vi "OtmMain.vi"() -> ()   [LabVIEW 2017]
doc: "This Continuous Measurement sample project is based on the Queued Message Handler template.\n\nThe Event Handling Loop generates messages based on user interface actions.\n\nThe Message Handling Loop processes messages generated by the Event Handling Loop, or by other messages. There are also Acquisition and Logging message handling loop subVIs, and a chart updating loop."
uses:
  Settings/Settings.ctl
  Acquisition/Hardware Configuration.ctl
  Acquisition/Signal Type.ctl
  Logging/Logging Configuration.ctl
  controls/UI Data.ctl
  controls/UI State.ctl
  support/Message Queue/Enqueue Message (Single).vi
  support/Message Queue/Enqueue Message (Array).vi
  <vilib>/Utility/error.llb/Error Cluster From Error Code.vi
  <vilib>/ErrorRing/Error Ring.xnode
  Logging/Logging.lvlib
  Settings/Settings.lvlib
  Acquisition/Acquisition.lvlib
  support/User Event - Stop/User Event - Stop.lvlib
  support/Message Queue/Message Queue.lvlib
  Settings/Settings Dialog.vi
panel:
  out "Data":waveform(dbl)[](graph)
  in  "Settings":bool
  in  "Start":bool
  in  "Stop":bool
  out "Status":string
  in  "Exit":bool
  # "Continuous Measurement Data Logger"
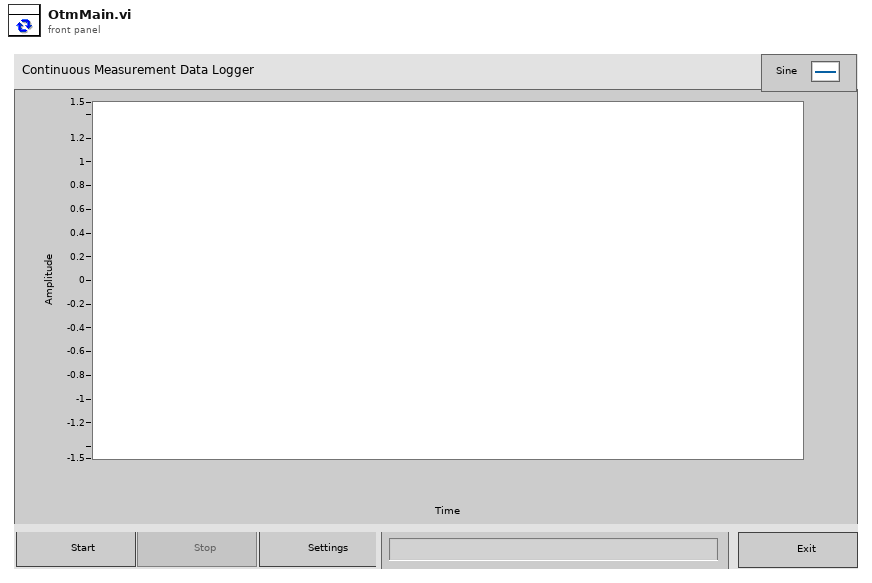
[diagram p1: front panel]
types:
  T1 = typedef "UI State.ctl" = enum16{"Idle", "Acquiring and Logging", "Waiting for Exit", "Waiting for Exit (Acq Stopped)", "Waiting for Exit (Log Stopped)", "Waiting for Stop", "Waiting for Stop (Acq Stopped)", "Waiting for Stop (Log Stopped)"}
  T2 = typedef "UI Data.ctl" = cluster{"Start Ref":refnum<vi>, "Stop Ref":refnum<vi>, "Settings Ref":refnum<vi>, "Exit Ref":refnum<vi>, "Status Ref":refnum<vi>, "Data Ref":refnum<vi>}
  T3 = typedef "Settings.lvlib/Settings.ctl" = cluster{"Hardware Configuration":T4, "Logging Configuration":T6}
  T4 = typedef "Acquisition.lvlib/Hardware Configuration.ctl" = cluster{"HW Refnum <Replace Me>":string, "Signal Type <Replace Me>":T5}
  T5 = typedef "Acquisition.lvlib/Signal Type.ctl" = enum16{"Sine Wave", "Square with Noise"}
  T6 = typedef "Logging.lvlib/Logging Configuration.ctl" = cluster{"Log File Base Path":path, "TDMS File Reference":refnum<k34>}
  T7 = typedef "Message Queue.lvlib/All Message Queues.ctl" = cluster{"UI":refnum<queue>, "Acquisition":refnum<queue>, "Logging":refnum<queue>}
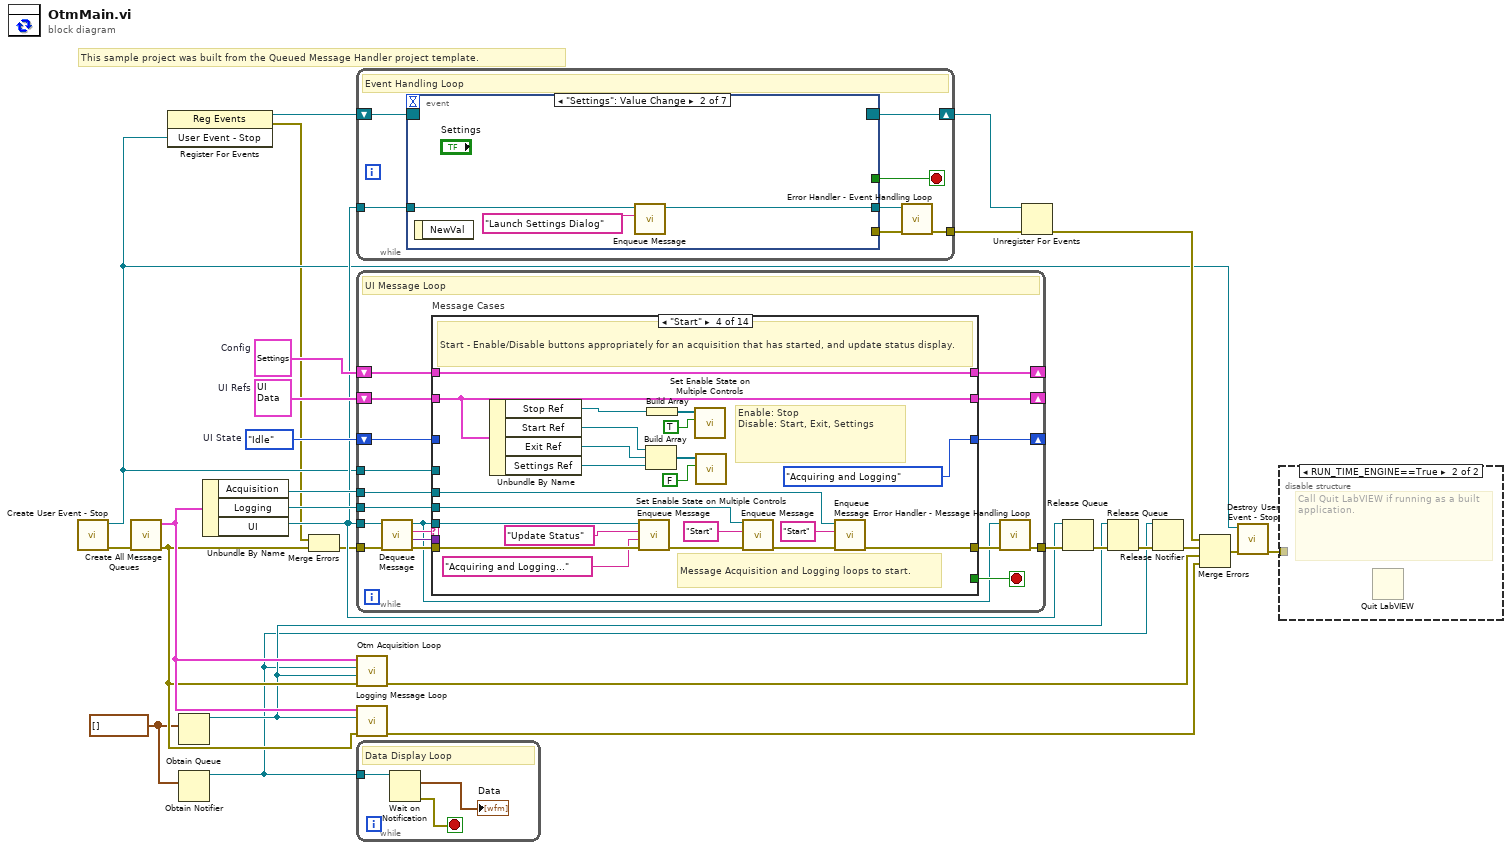
[diagram p0: block diagram]
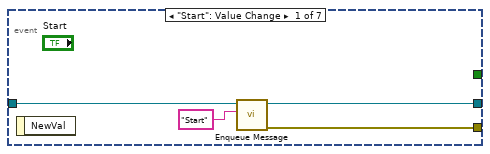
[diagram p3: hidden frame]
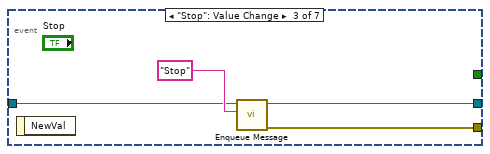
[diagram p4: hidden frame]
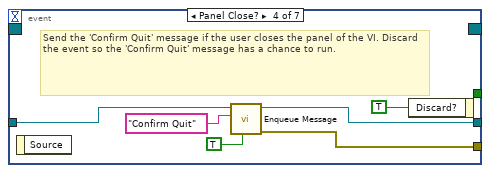
[diagram p5: hidden frame]
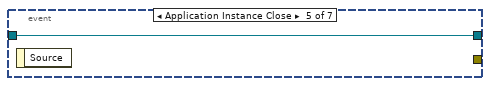
[diagram p6: hidden frame]
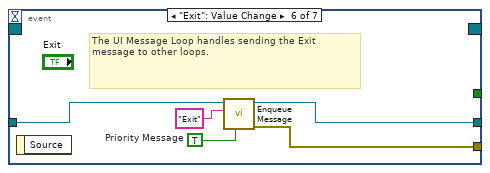
[diagram p7: hidden frame]
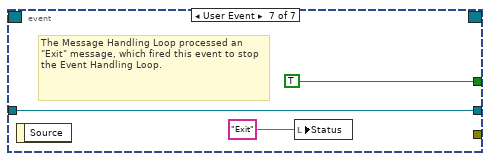
[diagram p8: hidden frame]
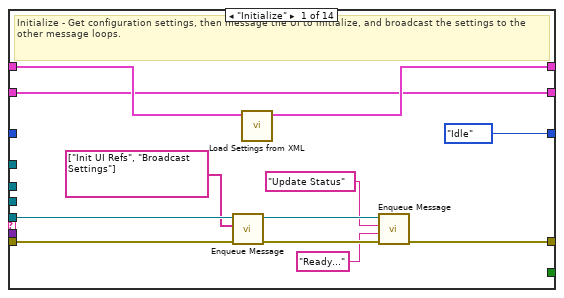
[diagram p9: hidden frame]
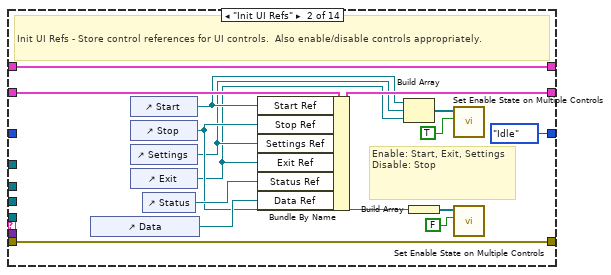
[diagram p10: hidden frame]
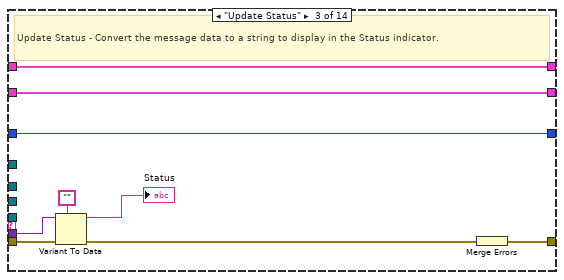
[diagram p11: hidden frame]
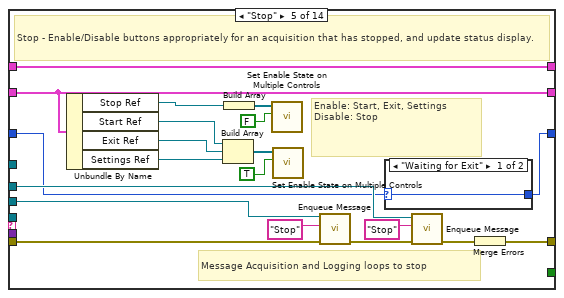
[diagram p12: hidden frame]
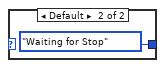
[diagram p13: hidden frame]
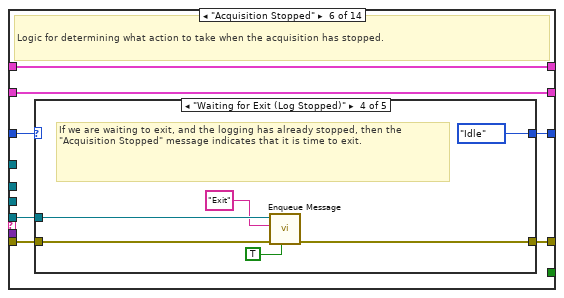
[diagram p14: hidden frame]
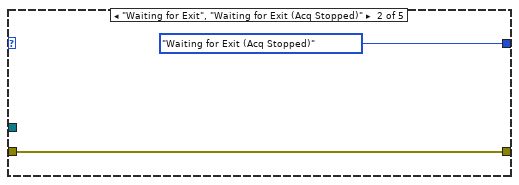
[diagram p16: hidden frame]
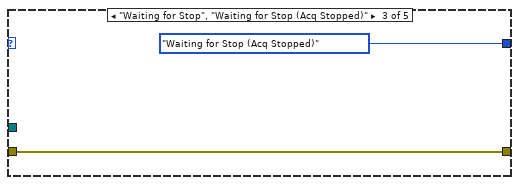
[diagram p17: hidden frame]
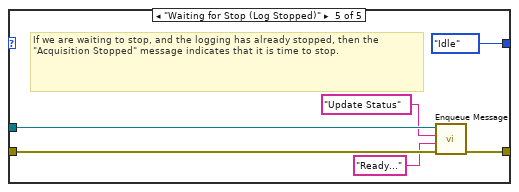
[diagram p18: hidden frame]
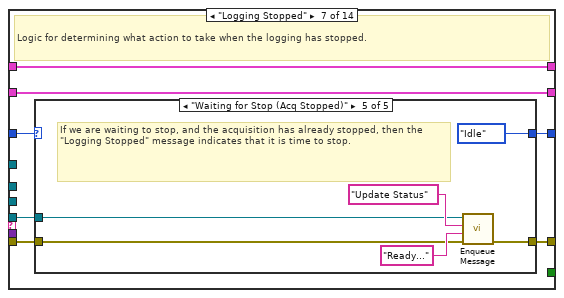
[diagram p19: hidden frame]
diagram:
  w14 = UI_State."Idle"  # UI State
  w5 = waveform(dbl)[] []
  w17 = T2 {"Start Ref"=refnum, "Stop Ref"=refnum, "Settings Ref"=refnum, "Exit Ref"=refnum, "Status Ref"=refnum, "Data Ref"=refnum}  # UI Refs
  w20 = T3 {"Hardware Configuration"={"HW Refnum <Replace Me>"="", "Signal Type <Replace Me>"=enum."Sine Wave"}, "Logging Configuration"={"Log File Base Path"=path "", "TDMS File Reference"=refnum}}  # Config
  # "This sample project was built from the Queued Message Handler project template."
  n1 = call "Create User Event - Stop.vi"() -> ("error out"=w24:errorcluster, "User Event - Stop"=w3:refnum<user-event>)  [unwired: 10 in]
  n2 = call "Create All Message Queues.vi"("error in (no error)"=w24) -> ("error out"=w21:errorcluster, "Message Queues out"=w23:T7)  [unwired: 9 in]
  n3 = register-events(w3) -> (reference out=w4:refnum<event-registration>, error out=w1:errorcluster)  [unwired: 2 in]
  n4 = Obtain Queue(element data type=w5) -> (queue out=w7:refnum<queue>)  [unwired: 4 in, 2 out]
  n5 = Obtain Notifier(notification data type=w5) -> (notifier out=w6:refnum<notifier>)  [unwired: 3 in, 2 out]
  n6 = Unbundle By Name(w23) -> ("Acquisition"=w16:refnum<queue>, "Logging"=w15:refnum<queue>, "UI"=w12:refnum<queue>)
  n7 = Merge Errors(w1, w21) -> (w2:errorcluster)
  n8 = while {
    tunnel: w12 -> [w33]
    tunnel: [w30] -> w26
    shift-right: [w32] -> w18
    shift-left: w4 -> [w34]
    stop <- w31 stop-if-true
    # "Event Handling Loop"
    n9 = event shown="[1] \"Settings\": Value Change" {
      selector: w34 -> [_ _ _ _ _ _ _]
      dyn-events: [_ _ _ _ _ _ _] -> w32
      timeout: _ -> [_ _ _ _ _ _ _]
      tunnel: [_ _ _ _ _ _ TRUE ("Discard?")] -> w31
      tunnel: w33 -> [w38 w40 w44 w49 w52 w54 w58]
      tunnel: [w36 _ w43 w47 _ w57 _] -> w29
      tunnel: [w35 w39 w42 w48 w52 w53 w58] -> w28
      event "Start": Value Change {
        n10 = event-data() -> ()  [unwired: 1 in, 1 out]
        n11 = call-poly "Enqueue Message.vi"("Message"="Start", "Message Queue"=w38) -> ("error out"=w36:errorcluster, "dup Message Queue"=w35:refnum<queue>)  [unwired: 8 in]
      }
      event "Settings": Value Change {
        n12 = event-data() -> ()  [unwired: 1 in, 1 out]
        n13 = call-poly "Enqueue Message.vi"("Message"="Launch Settings Dialog", "Message Queue"=w40) -> ("dup Message Queue"=w39:refnum<queue>)  [unwired: 8 in, 1 out]
      }
      event "Stop": Value Change {
        n14 = event-data() -> ()  [unwired: 1 in, 1 out]
        n15 = call-poly "Enqueue Message.vi"("Message"="Stop", "Message Queue"=w44) -> ("error out"=w43:errorcluster, "dup Message Queue"=w42:refnum<queue>)  [unwired: 8 in]
      }
      event Panel Close? {
        # "Send the 'Confirm Quit' message if the user closes the panel of the VI. Discard the event so the 'Confirm Quit' message has a chance to run."
        n16 = event-data() -> ()  [unwired: 1 in, 1 out]
        n17 = call-poly "Enqueue Message.vi"("Priority Message? (F)"=TRUE, "Message"="Confirm Quit", "Message Queue"=w49) -> ("error out"=w47:errorcluster, "dup Message Queue"=w48:refnum<queue>)  [unwired: 7 in]
        n18 = event-data("Discard?"=TRUE) -> ()  [unwired: 1 in, 1 out]
      }
      event Application Instance Close {
        n19 = event-data() -> ()  [unwired: 1 in, 1 out]
      }
      event "Exit": Value Change {
        w55 = TRUE  # Priority Message
        # "The UI Message Loop handles sending the Exit message to other loops."
        n20 = event-data() -> ()  [unwired: 1 in, 1 out]
        n21 = call-poly "Enqueue Message.vi"("Priority Message? (F)"=w55, "Message"="Exit", "Message Queue"=w54) -> ("error out"=w57:errorcluster, "dup Message Queue"=w53:refnum<queue>)  [unwired: 7 in]
      }
      event User Event {
        # "The Message Handling Loop processed an \"Exit\" message, which fired this event to stop the Event Handling Loop."
        n22 = event-data() -> ()  [unwired: 1 in, 1 out]
        n23 = local write "Status"("Exit" ("Exit String")) -> ()
      }
    }
    n24 = call "Error Handler - Event Handling Loop.vi"("error in (no error)"=w29, "Message Queue"=w28) -> ("dup error in"=w30:errorcluster)  [unwired: 8 in, 1 out]
  }
  n25 = while {
    tunnel: w12 -> [w72]
    tunnel: w3 -> [w77]
    shift-right: [w71] -> _
    shift-left: w20 -> [w70]
    shift-right: [w68] -> _
    shift-left: w17 -> [w69]
    tunnel: w16 -> [w67]
    tunnel: w15 -> [w66]
    shift-right: [w61] -> _
    shift-left: w14 -> [w62]
    tunnel: w2 -> [w76]
    tunnel: [w65] -> w27
    stop <- w78 stop-if-true
    # "UI Message Loop"
    n26 = call "Dequeue Message.vi"("error in (no error)"=w76, "Message Queue"=w72) -> ("error out"=w75:errorcluster, "Message Data"=w73:variant, "Message"=w74:string, "dup Message Queue"=w63:refnum<queue>)  [unwired: 6 in]
    n27 = case "Message Cases" shown="\"Start\"" w74 {
      selector: w74 -> [_ _ _ _ _ _ _ _ _ _ _ _ _ w294]
      tunnel: w63 -> [w82 _ _ w136 _ w161 w186 _ w226 _ w247 _ _ _]
      tunnel: w75 -> [w81 w105 w113 w135 w155 w162 w187 w214 w228 w235 w246 w275 w292 _]
      tunnel: [w86 w105 w114 w118 w156 w159 w184 w220 w221 w238 w245 w285 w291 w293] -> w64
      tunnel: [_ _ _ _ _ _ _ _ _ _ _ TRUE _ _] -> w78
      tunnel: w73 -> [_ _ w112 _ _ _ _ _ _ w239 _ w273 _ _]
      tunnel: w77 -> [_ _ _ _ _ _ _ _ _ _ _ w286 _ _]
      tunnel: [w89 w104 w108 w134 w154 w165 w190 w218 w225 w243 w250 w284 w290 w297] -> w71
      tunnel: w70 -> [w90 w104 w108 w134 w154 w165 w190 w218 w229 w243 w250 w284 w290 w297]
      tunnel: w69 -> [w83 w103 w107 w131 w153 w164 w189 w212 w223 w242 w249 w283 w289 w296]
      tunnel: [w83 w100 w107 w131 w153 w164 w189 w212 w223 w242 w249 w283 w289 w296] -> w68
      tunnel: w67 -> [_ _ _ w117 w140 _ _ w211 _ _ _ w282 _ _]
      tunnel: w66 -> [_ _ _ w120 w143 _ _ w210 _ _ _ w281 _ _]
      tunnel: w62 -> [_ _ w106 _ w137 w163 w188 w209 w222 w237 w248 _ w288 w295]
      tunnel: [UI_State."Idle" ("UI State") UI_State."Idle" ("UI State") w106 UI_State."Acquiring and Logging" ("UI State") w138 w160 w185 w209 w222 w237 w244 UI_State."Idle" ("UI State") w288 w295] -> w61
      frame "Initialize" {
        # "Initialize - Get configuration settings, then message the UI to initialize, and broadcast the settings to the other message loops."
        n28 = call-poly "Enqueue Message.vi"("error in (no error)"=w81, "Message Array"=string[] ["Init UI Refs", "Broadcast Settings"], "Message Queue"=w82) -> ("error out"=w88:errorcluster, "dup Message Queue"=w87:refnum<queue>)  [unwired: 7 in]
        n29 = call "Load Settings from XML.vi"("Settings in"=w90) -> ("Settings out"=w89:T3)  [unwired: 9 in, 1 out]
        n30 = call-poly "Enqueue Message.vi"("error in (no error)"=w88, "Message Data"="Ready..." ("Ready..."), "Message"="Update Status", "Message Queue"=w87) -> ("error out"=w86:errorcluster)  [unwired: 6 in, 1 out]
      }
      frame "Init UI Refs" {
        # "Enable: Start, Exit, Settings\nDisable: Stop"
        # "Init UI Refs - Store control references for UI controls.  Also enable/disable controls appropriately."
        n31 = control-ref of="Data"() -> (w101:refnum<vi>)
        n32 = control-ref of="Start"() -> (w94:refnum<vi>)
        n33 = control-ref of="Stop"() -> (w95:refnum<vi>)
        n34 = control-ref of="Settings"() -> (w93:refnum<vi>)
        n35 = control-ref of="Exit"() -> (w92:refnum<vi>)
        n36 = control-ref of="Status"() -> (w102:refnum<vi>)
        n37 = Bundle By Name(cluster=w103, "Start Ref"=w94, "Stop Ref"=w95, "Settings Ref"=w93, "Exit Ref"=w92, "Status Ref"=w102, "Data Ref"=w101) -> (w100:T2)
        n38 = Build Array(w94, w93, w92) -> (w98:refnum<vi>[])
        n39 = Build Array(w95) -> (w97:refnum<vi>[])
        n40 = call "Set Enable State on Multiple Controls.vi"("Enable?"=TRUE, "Controls"=w98) -> ()  [unwired: 10 in]
        n41 = call "Set Enable State on Multiple Controls.vi"("Enable?"=FALSE, "Controls"=w97) -> ()  [unwired: 10 in]
      }
      frame "Update Status" {
        # "Update Status - Convert the message data to a string to display in the Status indicator."
        n42 = Variant To Data(error in=w113, type="", Variant=w112) -> (data=→"Status":string, error out=w110:errorcluster)
        n43 = Merge Errors(w110) -> (w114:errorcluster)
      }
      frame "Start" {
        # "Message Acquisition and Logging loops to start."
        # "Enable: Stop\nDisable: Start, Exit, Settings"
        # "Start - Enable/Disable buttons appropriately for an acquisition that has started, and update status display."
        n44 = Unbundle By Name(w131) -> ("Stop Ref"=w126:refnum<vi>, "Start Ref"=w125:refnum<vi>, "Exit Ref"=w124:refnum<vi>, "Settings Ref"=w123:refnum<vi>)
        n45 = call-poly "Enqueue Message.vi"("error in (no error)"=w135, "Message Data"="Acquiring and Logging..." ("Acquiring and Logging..."), "Message"="Update Status", "Message Queue"=w136) -> ("error out"=w122:errorcluster)  [unwired: 6 in, 1 out]
        n46 = Build Array(w125, w124, w123) -> (w129:refnum<vi>[])
        n47 = Build Array(w126) -> (w128:refnum<vi>[])
        n48 = call "Set Enable State on Multiple Controls.vi"("Enable?"=TRUE, "Controls"=w128) -> ()  [unwired: 10 in]
        n49 = call "Set Enable State on Multiple Controls.vi"("Enable?"=FALSE, "Controls"=w129) -> ()  [unwired: 10 in]
        n50 = call-poly "Enqueue Message.vi"("error in (no error)"=w122, "Message"="Start", "Message Queue"=w120) -> ("error out"=w119:errorcluster)  [unwired: 7 in, 1 out]
        n51 = call-poly "Enqueue Message.vi"("error in (no error)"=w119, "Message"="Start", "Message Queue"=w117) -> ("error out"=w118:errorcluster)  [unwired: 7 in, 1 out]
      }
      frame "Stop" {
        # "Message Acquisition and Logging loops to stop"
        # "Enable: Start, Exit, Settings\nDisable: Stop"
        # "Stop - Enable/Disable buttons appropriately for an acquisition that has stopped, and update status display."
        n52 = Unbundle By Name(w153) -> ("Stop Ref"=w148:refnum<vi>, "Start Ref"=w147:refnum<vi>, "Exit Ref"=w146:refnum<vi>, "Settings Ref"=w145:refnum<vi>)
        n53 = Build Array(w147, w146, w145) -> (w151:refnum<vi>[])
        n54 = Build Array(w148) -> (w150:refnum<vi>[])
        n55 = call "Set Enable State on Multiple Controls.vi"("Enable?"=FALSE, "Controls"=w150) -> ()  [unwired: 10 in]
        n56 = call "Set Enable State on Multiple Controls.vi"("Enable?"=TRUE, "Controls"=w151) -> ()  [unwired: 10 in]
        n57 = call-poly "Enqueue Message.vi"("error in (no error)"=w155, "Message"="Stop", "Message Queue"=w143) -> ("error out"=w142:errorcluster)  [unwired: 7 in, 1 out]
        n58 = case shown="\"Waiting for Exit\"" w137 {
          selector: w137 -> [w157 _]
          tunnel: [w157 UI_State."Waiting for Stop" ("UI State")] -> w138
          frame "Waiting for Exit" {
          }
          frame Default {
          }
        }
        n59 = call-poly "Enqueue Message.vi"("error in (no error)"=w142, "Message"="Stop", "Message Queue"=w140) -> ("error out"=w141:errorcluster)  [unwired: 7 in, 1 out]
        n60 = Merge Errors(w141) -> (w156:errorcluster)
      }
      frame "Acquisition Stopped" {
        # "Logic for determining what action to take when the acquisition has stopped."
        n61 = case shown="\"Waiting for Exit (Log Stopped)\"" w163 {
          selector: w163 -> [w167 _ _ _ _]
          tunnel: w162 -> [w166 w169 w171 w177 w183]
          tunnel: w161 -> [_ _ _ w175 w180]
          tunnel: [w167 UI_State."Waiting for Exit (Acq Stopped)" ("UI State") UI_State."Waiting for Stop (Acq Stopped)" ("UI State") UI_State."Idle" ("UI State") UI_State."Idle" ("UI State")] -> w160
          tunnel: [w166 w169 w171 w176 w181] -> w159
          frame Default {
          }
          frame "Waiting for Exit", "Waiting for Exit (Acq Stopped)" {
          }
          frame "Waiting for Stop", "Waiting for Stop (Acq Stopped)" {
          }
          frame "Waiting for Exit (Log Stopped)" {
            # "If we are waiting to exit, and the logging has already stopped, then the \"Acquisition Stopped\" message indicates that it is time to exit."
            n62 = call-poly "Enqueue Message.vi"("Priority Message? (F)"=TRUE, "error in (no error)"=w177, "Message"="Exit", "Message Queue"=w175) -> ("error out"=w176:errorcluster)  [unwired: 6 in, 1 out]
          }
          frame "Waiting for Stop (Log Stopped)" {
            # "If we are waiting to stop, and the logging has already stopped, then the \"Acquisition Stopped\" message indicates that it is time to stop."
            n63 = call-poly "Enqueue Message.vi"("error in (no error)"=w183, "Message Data"="Ready..." ("Ready..."), "Message"="Update Status", "Message Queue"=w180) -> ("error out"=w181:errorcluster)  [unwired: 6 in, 1 out]
          }
        }
      }
      frame "Logging Stopped" {
        # "Logic for determining what action to take when the logging has stopped."
        n64 = case shown="\"Waiting for Stop (Acq Stopped)\"" w188 {
          selector: w188 -> [w192 _ _ _ _]
          tunnel: w187 -> [w191 w194 w196 w202 w205]
          tunnel: w186 -> [_ _ _ w200 w204]
          tunnel: [w192 UI_State."Waiting for Exit (Log Stopped)" ("UI State") UI_State."Waiting for Stop (Log Stopped)" ("UI State") UI_State."Idle" ("UI State") UI_State."Idle" ("UI State")] -> w185
          tunnel: [w191 w194 w196 w201 w203] -> w184
          frame Default {
          }
          frame "Waiting for Exit", "Waiting for Exit (Log Stopped)" {
          }
          frame "Waiting for Stop", "Waiting for Stop (Log Stopped)" {
          }
          frame "Waiting for Exit (Acq Stopped)" {
            # "If we are waiting to exit, and the acquisition has already stopped, then the \"Logging Stopped\" message indicates that it is time to exit."
            n65 = call-poly "Enqueue Message.vi"("Priority Message? (F)"=TRUE, "error in (no error)"=w202, "Message"="Exit", "Message Queue"=w200) -> ("error out"=w201:errorcluster)  [unwired: 6 in, 1 out]
          }
          frame "Waiting for Stop (Acq Stopped)" {
            # "If we are waiting to stop, and the acquisition has already stopped, then the \"Logging Stopped\" message indicates that it is time to stop."
            n66 = call-poly "Enqueue Message.vi"("error in (no error)"=w205, "Message Data"="Ready..." ("Ready..."), "Message"="Update Status", "Message Queue"=w204) -> ("error out"=w203:errorcluster)  [unwired: 6 in, 1 out]
          }
        }
      }
      frame "Broadcast settings" {
        w213 = "Update Settings" ("Message")
        # "Broadcast settings - Send the 'Update Settings' message to the Logging and Acquisition message loops."
        n67 = Unbundle By Name(w218) -> ("Hardware Configuration"=w217:T4, "Logging Configuration"=w216:T6)
        n68 = call-poly "Enqueue Message.vi"("Message Data"=w217, "Message"=w213, "Message Queue"=w211) -> ("error out"=w219:errorcluster)  [unwired: 7 in, 1 out]
        n69 = call-poly "Enqueue Message.vi"("error in (no error)"=w219, "Message Data"=w216, "Message"=w213, "Message Queue"=w210) -> ("error out"=w215:errorcluster)  [unwired: 6 in, 1 out]
        n70 = Merge Errors(w215, w214) -> (w220:errorcluster)
      }
      frame "Launch Settings Dialog" {
        # "Launch Settings Dialog - Launch the Settings Dialog when the user clicks the 'Settings' button."
        n71 = call-by-ref "?"("error in (no error)"=w228, "Settings in"=w229) -> ("error out"=w224:errorcluster, "Cancelled?"=w227:bool, "Settings out"=w225:T3)  [unwired: 8 in, 3 out]
        n72 = case shown="False" w227 {
          tunnel: w226 -> [w233 _]
          tunnel: w224 -> [w232 w234]
          tunnel: [w231 w234] -> w221
          frame False {
            n73 = call-poly "Enqueue Message.vi"("error in (no error)"=w232, "Message"="Broadcast Settings", "Message Queue"=w233) -> ("error out"=w231:errorcluster)  [unwired: 7 in, 1 out]
          }
          frame True {
          }
        }
      }
      frame "Error" {
        # "Error - Display an error dialog. This message is sent by the \"Error Handler\" VIs at the end of other loops in this application."
        n74 = Variant To Data(error in=w235, type=errorcluster {"status"=FALSE, "code"=0, "source"=""} ("error constant"), Variant=w239) -> (data=w236:errorcluster, error out=w240:errorcluster)
        n75 = call <vilib>:"Simple Error Handler.vi"("error in (no error)"=w236) -> ()  [unwired: 4 in, 5 out]
        n76 = Merge Errors(w240) -> (w238:errorcluster)
      }
      frame "Confirm Quit" {
        # "Confirm Quit - Message that can confirm whether or not the user wants to exit the application."
        n77 = case shown="\"Acquiring and Logging\"" w248 {
          tunnel: w247 -> [w256 w260]
          tunnel: w246 -> [w255 w259]
          tunnel: [w254 w258] -> w245
          tunnel: [UI_State."Idle" ("UI State") w257] -> w244
          frame Default {
            # "If 'Confirm Quit' comes in while the system is idle, there is no need for a confirmation message."
            n78 = call-poly "Enqueue Message.vi"("Priority Message? (F)"=TRUE, "error in (no error)"=w255, "Message"="Exit", "Message Queue"=w256) -> ("error out"=w254:errorcluster)  [unwired: 6 in, 1 out]
          }
          frame "Acquiring and Logging" {
            n79 = Two Button Dialog(message="Are you sure you want to quit while the acquisition is running?" ("Confirm Quit Message"), 1:"No" ("No"), 2:"Yes" ("Yes")) -> (T button?=w261:bool)
            n80 = case shown="True" w261 {
              tunnel: w260 -> [_ w270]
              tunnel: w259 -> [w266 w271]
              tunnel: [w266 w269] -> w258
              tunnel: [UI_State."Acquiring and Logging" ("UI State") UI_State."Waiting for Exit" ("UI State")] -> w257
              frame False {
                # "User did not want to quit."
              }
              frame True {
                n81 = call-poly "Enqueue Message.vi"("error in (no error)"=w271, "Message"="Stop", "Message Queue"=w270) -> ("error out"=w269:errorcluster)  [unwired: 7 in, 1 out]
              }
            }
          }
        }
      }
      frame "Exit" {
        w277 = TRUE ("Priority Message? (F)")
        w278 = "Exit" ("Message")
        # "Popup an error dialog if 'Exit' was called as a result of an error."
        # "Stop the VI"
        # "Exit - Send Exit messages to the Acquisition and Logging loops, and fire the user event to stop the Event Handling Loop."
        n82 = Variant To Data(type=errorcluster {"status"=FALSE, "code"=0, "source"=""} ("error constant"), Variant=w273) -> (data=w272:errorcluster)  [unwired: 1 in, 1 out]
        n83 = call <vilib>:"Simple Error Handler.vi"("error in (no error)"=w272) -> ()  [unwired: 4 in, 5 out]
        n84 = call-poly "Enqueue Message.vi"("Priority Message? (F)"=w277, "error in (no error)"=w275, "Message"=w278, "Message Queue"=w282) -> ("error out"=w279:errorcluster)  [unwired: 6 in, 1 out]
        n85 = call-poly "Enqueue Message.vi"("Priority Message? (F)"=w277, "error in (no error)"=w279, "Message"=w278, "Message Queue"=w281) -> ("error out"=w276:errorcluster)  [unwired: 6 in, 1 out]
        n86 = call "Fire User Event - Stop.vi"("error in (no error)"=w276, "User Event - Stop"=w286) -> ("error out"=w285:errorcluster)  [unwired: 9 in]
      }
      frame "---Copy This Frame---" {
        # "Duplicate this frame when creating new messages.  Change this comment in the duplicated frame to describe this message."
        n87 = Merge Errors(w292) -> (w291:errorcluster)
      }
      frame Default {
        # "'Default' case only runs if there is a message that isn't defined in any of the other cases.  Output a programming error."
        n88 = xnode "Error Ring"("parameter 0"=w294) -> ("error out"=w293:errorcluster)
      }
    }
    n89 = call "Error Handler - Message Handling Loop.vi"("error in (no error)"=w64, "Message Queue"=w63) -> ("dup error in"=w65:errorcluster)  [unwired: 8 in, 1 out]
  }
  n90 = call "Otm Acquisition Loop.vi"("error in (no error)"=w21, "Data Queue"=w7, "Data Notifier"=w6, "Message Queues"=w23) -> ("error out"=w25:errorcluster)  [unwired: 7 in]
  n91 = call "Logging Message Loop.vi"("error in (no error)"=w21, "Data Queue"=w7, "Message Queues"=w23) -> ("error out"=w22:errorcluster)  [unwired: 8 in]
  n92 = while "Data Display Loop" {
    tunnel: w6 -> [w307]
    stop <- w305 stop-if-true
    # "Data Display Loop"
    n93 = Wait on Notification(notifier=w307) -> (notification=→"Data":waveform(dbl)[], error out=w305:errorcluster)  [unwired: 3 in, 2 out]
  }
  n94 = Unregister For Events(event registration refnum=w18, error in=w26) -> (error out=w19:errorcluster)
  n95 = Release Queue(queue=w12, error in (no error)=w27) -> (error out=w10:errorcluster)  [unwired: 1 in, 2 out]
  n96 = Release Queue(queue=w7, error in (no error)=w10) -> (error out=w9:errorcluster)  [unwired: 1 in, 2 out]
  n97 = Release Notifier(notifier=w6, error in (no error)=w9) -> (error out=w8:errorcluster)  [unwired: 1 in, 2 out]
  n98 = Merge Errors(w19, w8, w25, w22) -> (w13:errorcluster)
  n99 = call "Destroy User Event - Stop.vi"("error in (no error)"=w13, "User Event - Stop"=w3) -> ("error out"=w11:errorcluster)  [unwired: 9 in]
  n100 = disable-structure shown="RUN_TIME_ENGINE==True" {
    disable-tunnel: w11 -> [_ _]
    frame condition #0 (active) {
    }
    frame condition #1 {
      # "Call Quit LabVIEW if running as a built application."
      n101 = Quit LabVIEW() -> ()  [unwired: 1 in]
    }
  }
